vi "Publisher Cluster to device cluster.vi"(11 "publisher cluster":T1) -> (3 "Device cluster":T3)   [LabVIEW 2013]
uses:
  dataCluster.ctl
  <vilib>/vision/Image Controls.llb/IMAQ Image.ctl
  DataQueueTypeDef.ctl
  PolyWrite/String.vi
  PolyWrite/error.vi
  PolyWrite/U32.vi
  PolyWrite/Path.vi
  PolyWrite/I32.vi
  PolyWrite/Boolean.vi
  PolyWrite/I32ref.vi
panel:
  out "Image Storage":string[](array[string])
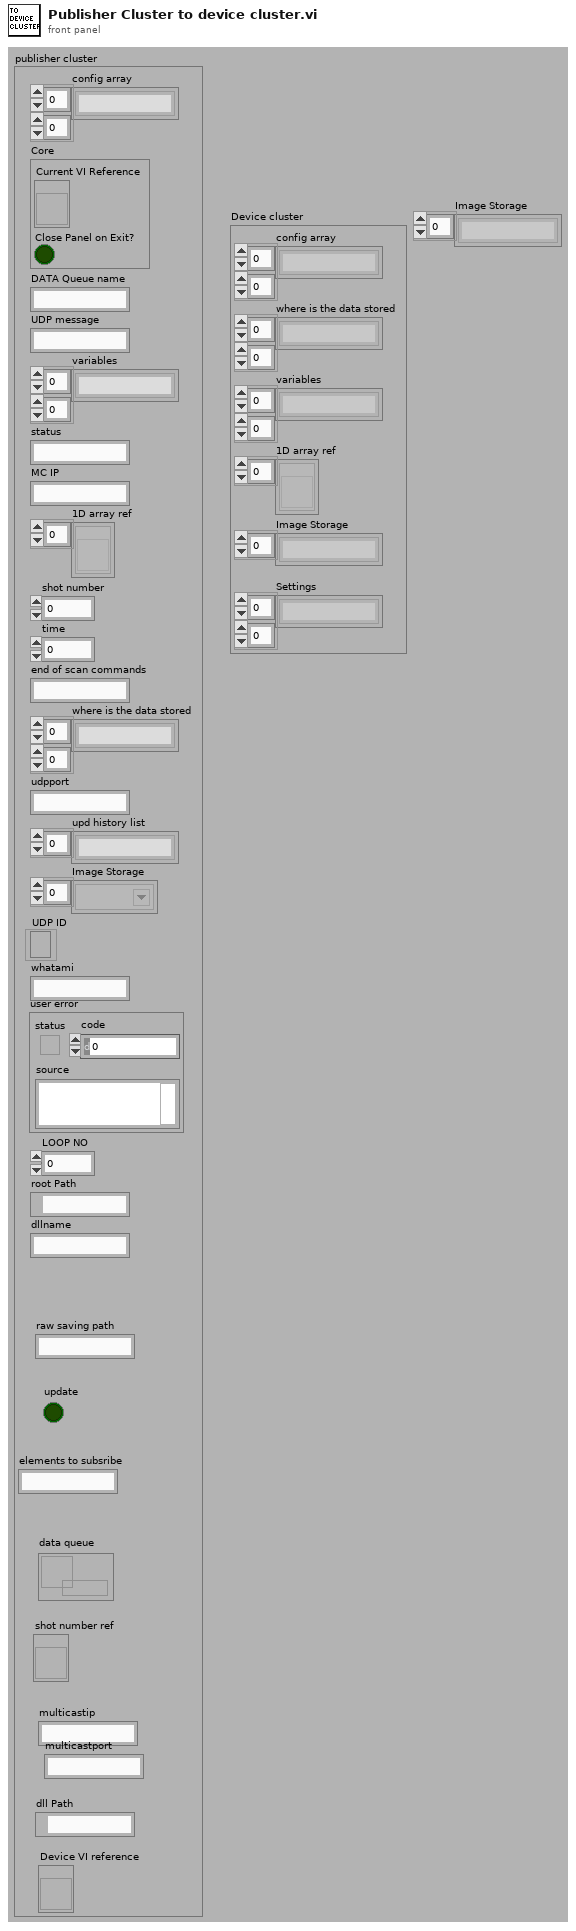
[diagram p1: front panel]
types:
  T1 = typedef "dataCluster.ctl" = cluster{"config array":string[][], "Core":cluster{"Current VI Reference":refnum<vi>, "Close Panel on Exit?":bool}, "DATA Queue name":string, "UDP message":string, "variables":string[][], "status":string, "MC IP":string, "1D array ref":refnum<vi>[], "shot number":i32, "time":u32, "end of scan commands":string, "where is the data stored":string[][], "udpport":string, "upd history list":string[], "Image Storage":T2[], "UDP ID":refnum<k16>, "whatami":string, "user error":errorcluster, "LOOP NO":u32, "root Path":path, "dllname":string, "raw saving path":string, "update":bool, "elements to subsribe":string, "data queue":refnum<queue>, "shot number ref":refnum<vi>, "multicastip":string, "multicastport":string, "dll Path":path, "Device VI reference":refnum<vi>}
  T2 = typedef "IMAQ Image.ctl" = refnum<image>
  T3 = cluster{"config array":string[][], "where is the data stored":string[][], "variables":string[][], "1D array ref":refnum<vi>[], "Image Storage":string[], "Settings":string[][]}
  T4 = cluster{"config array":string[][], "where is the data stored":string[][], "variables":string[][], "1D array ref":refnum<vi>[], string[], "array out":string[][]}
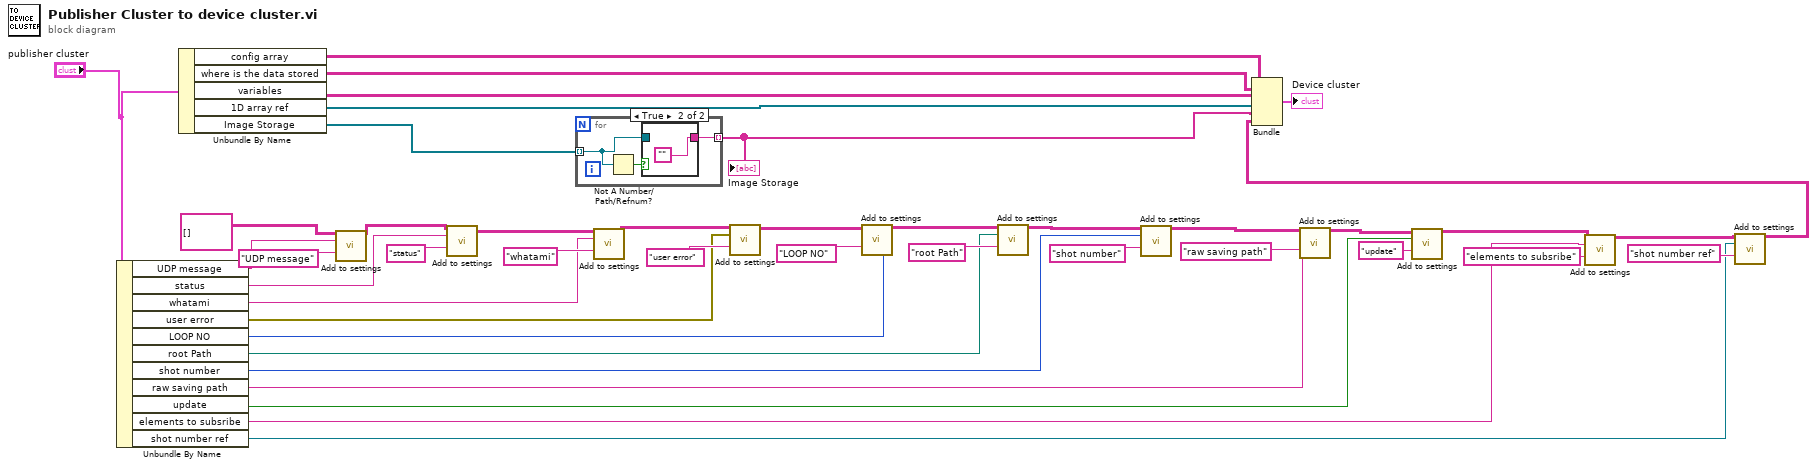
[diagram p0: block diagram]
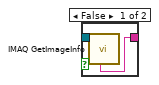
[diagram p2: hidden frame]
diagram:
  n1 = Unbundle By Name("publisher cluster") -> ("UDP message"=w17:string, "status"=w22:string, "whatami"=w39:string, "user error"=w36:errorcluster, "LOOP NO"=w33:u32, "root Path"=w30:path, "shot number"=w21:i32, "raw saving path"=w12:string, "update"=w9:bool, "elements to subsribe"=w5:string, "shot number ref"=w2:refnum<vi>)
  n2 = Unbundle By Name("publisher cluster") -> ("config array"=w27:string[][], "where is the data stored"=w26:string[][], "variables"=w25:string[][], "1D array ref"=w24:refnum<vi>[], "Image Storage"=w23:T2[])
  n3 = call-poly "Add to settings.vi"("array in"=string[][] [], "string"=w17, "Variable Name"="UDP message" ("string")) -> ("array out"=w18:string[][])  [unwired: 11 in, 1 out]
  n4 = call-poly "Add to settings.vi"("array in"=w18, "string"=w22, "Variable Name"="status" ("string")) -> ("array out"=w40:string[][])  [unwired: 11 in, 1 out]
  n5 = for {
    tunnel: w23 -> [w44] mode=indexing
    tunnel: [w45] -> w15 mode=indexing
    n6 = Not A Number/Path/Refnum?(number/path/refnum=w44) -> (NaN/Path/Refnum?=w43:bool)
    n7 = case shown="True" w43 {
      tunnel: [w47 ""] -> w45
      tunnel: w44 -> [w46 _]
      frame False {
        n8 = call "IMAQ GetImageInfo"("Image"=w46) -> ("Image Name"=w47:string)  [unwired: 3 in, 7 out]
      }
      frame True {
      }
    }
  }
  "Image Storage" <- w15
  n9 = call-poly "Add to settings.vi"("array in"=w40, "string"=w39, "Variable Name"="whatami") -> ("array out"=w38:string[][])  [unwired: 11 in, 1 out]
  n10 = call-poly "Add to settings.vi"("array in"=w38, "error"=w36, "Variable Name"="user error") -> ("array out"=w34:string[][])  [unwired: 11 in, 1 out]
  n11 = call-poly "Add to settings.vi"("array in"=w34, "LOOP NO"=w33, "Variable Name"="LOOP NO") -> ("array out"=w31:string[][])  [unwired: 11 in, 1 out]
  n12 = call-poly "Add to settings.vi"("array in"=w31, "Path"=w30, "Variable Name"="root Path") -> ("array out"=w28:string[][])  [unwired: 11 in, 1 out]
  n13 = call-poly "Add to settings.vi"("array in"=w28, "Anything"=w21, "Variable Name"="shot number") -> ("array out"=w8:string[][])  [unwired: 11 in, 1 out]
  n14 = call-poly "Add to settings.vi"("array in"=w8, "string"=w12, "Variable Name"="raw saving path") -> ("array out"=w10:string[][])  [unwired: 11 in, 1 out]
  n15 = call-poly "Add to settings.vi"("array in"=w10, "Boolean"=w9, "Variable Name"="update") -> ("array out"=w6:string[][])  [unwired: 11 in, 1 out]
  n16 = call-poly "Add to settings.vi"("array in"=w6, "string"=w5, "Variable Name"="elements to subsribe") -> ("array out"=w4:string[][])  [unwired: 11 in, 1 out]
  n17 = call-poly "Add to settings.vi"("array in"=w4, "I32ref"=w2, "Variable Name"="shot number ref") -> ("array out"=w1:string[][])  [unwired: 11 in, 1 out]
  n18 = Bundle("config array"=w27, "where is the data stored"=w26, "variables"=w25, "1D array ref"=w24, w15, "array out"=w1) -> (→"Device cluster":T4)  [unwired: 1 in]
